vi "ETag String.vi"(10 "Weak":bool, 11 "ETag":string) -> (3 "ETag Value":string)   [LabVIEW 2020, in "HTTP Utils.lvlib"]
uses:
  HTTP Utils.lvlib
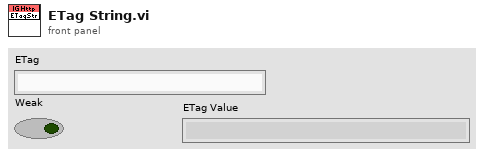
[diagram p1: front panel]
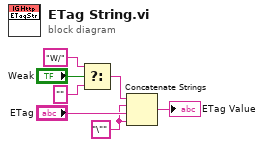
[diagram p0: block diagram]
diagram:
  w4 = "\""
  n1 = Select(t="W/", s="Weak", f="") -> (s? t:f=w2:string)
  n2 = Concatenate Strings(w2, w4, "ETag", w4) -> (→"ETag Value":string)
